vi "Delete_Fake_Dots_From_Array([-1,-1...]).vi"(2 "error IN":errorcluster, 3 "[IN] Source Array":dbl[][](array[numeric])) -> (0 "error OUT":errorcluster, 1 "[OUT] Filtered Array (X,Y,dX,dY)":dbl[][](array[numeric]))   [LabVIEW 2017]
doc: "Getting rid of deleted displacements (-1,-1,...)"
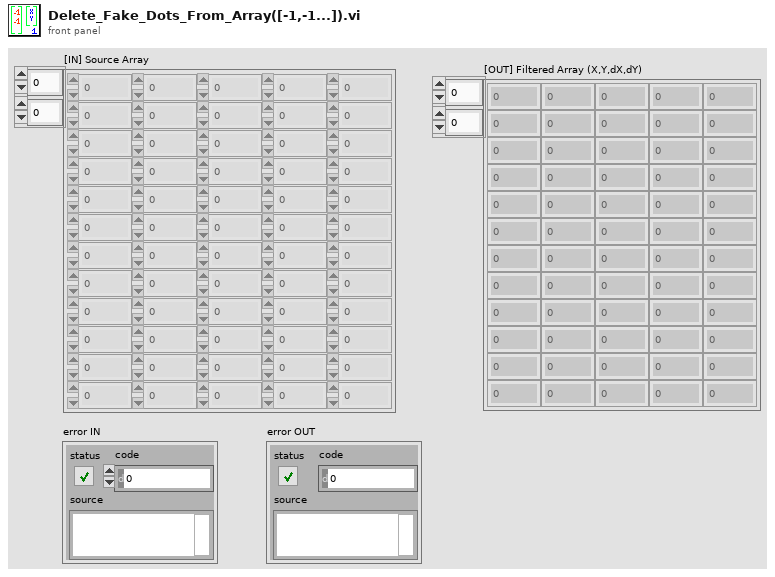
[diagram p1: front panel]
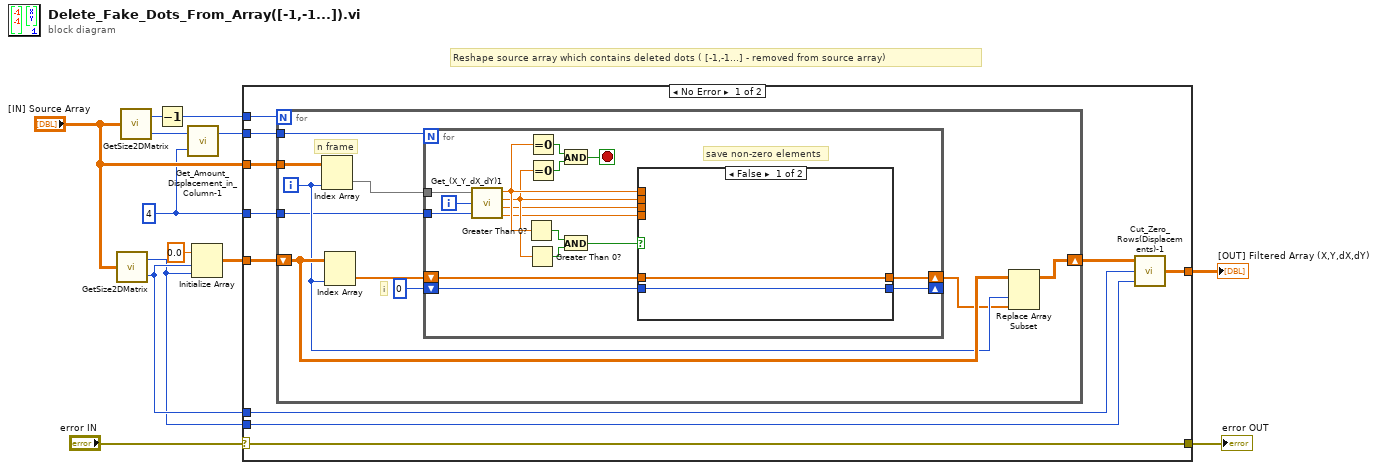
[diagram p0: block diagram]
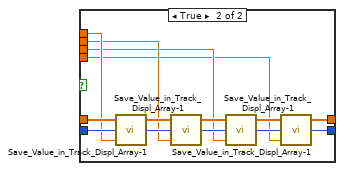
[diagram p2: hidden frame]
diagram:
  w3 = 4 ("y")
  # "Reshape source array which contains deleted dots ( [-1,-1...] - removed from source array)"
  n1 = call "GetSize2DMatrix.vi"("Array IN (2D)"="[IN] Source Array") -> ("# Cols"=w7:i32, "# Rows"=w8:i32)
  n2 = call "GetSize2DMatrix.vi"("Array IN (2D)"="[IN] Source Array") -> ("# Cols"=w13:i32, "# Rows"=w5:i32)
  n3 = Decrement(x=w13) -> (x-1=w12:i32)
  n4 = call "Get_Amount_Displacement_in_Column-1.vi"("multiplier"=w3, "# Rows"=w5) -> ("Displ amount"=w4:i32)  [unwired: 1 out]
  n5 = Initialize Array(0.0 ("element"), w8, w7) -> (w9:dbl[][])
  n6 = case shown="No Error" "error IN" {
    selector: "error IN" -> [w14 w67]
    tunnel: w12 -> [w23 _]
    tunnel: "[IN] Source Array" -> [w22 _]
    tunnel: w9 -> [w21 w68]
    tunnel: w8 -> [w19 _]
    tunnel: w7 -> [w18 _]
    tunnel: [w17 w68] -> w6
    tunnel: w4 -> [w16 _]
    tunnel: w3 -> [w15 _]
    tunnel: [w14 w67] -> w1
    frame No Error {
      n7 = for {
        N: w23 -> [_]
        tunnel: w22 -> [w33]
        shift-right: [w29] -> w20
        shift-left: w21 -> [w30]
        tunnel: w16 -> [w25]
        tunnel: w15 -> [w24]
        i -> [w28]
        # "i"
        # "n frame"
        n8 = Index Array(array=w33, index (col)=w28) -> (element=w31:dbl[])  [unwired: 1 in]
        n9 = Index Array(array=w30, index (col)=w28) -> (element=w26:dbl[])  [unwired: 1 in]
        n10 = for {
          N: w25 -> [_]
          tunnel: w31 -> [w50]
          tunnel: w24 -> [w48]
          shift-right: [w34] -> w27
          shift-left: w26 -> [w41]
          shift-right: [w35] -> _
          shift-left: 0 -> [w40]
          i -> [w49]
          stop <- w45 stop-if-true
          # "save non-zero elements"
          n11 = call "Get_(X_Y_dX_dY)1.vi"("(X,Y,dX,dY)"=w50, "index"=w49, "multiplier"=w48) -> ("X"=w39:dbl, "Y"=w38:dbl, "dX"=w37:dbl, "dY"=w36:dbl)
          n12 = Greater Than 0?(x=w39) -> (x > 0?=w44:bool)
          n13 = Greater Than 0?(x=w38) -> (x > 0?=w43:bool)
          n14 = Equal To 0?(x=w39) -> (x = 0?=w47:bool)
          n15 = Equal To 0?(x=w38) -> (x = 0?=w46:bool)
          n16 = And(x=w47, y=w46) -> (x .and. y?=w45:bool)
          n17 = And(x=w44, y=w43) -> (x .and. y?=w42:bool)
          n18 = case shown="False" w42 {
            tunnel: w41 -> [w52 w66]
            tunnel: w40 -> [w51 w65]
            tunnel: w39 -> [_ w64]
            tunnel: w38 -> [_ w61]
            tunnel: w37 -> [_ w58]
            tunnel: w36 -> [_ w55]
            tunnel: [w51 w53] -> w35
            tunnel: [w52 w54] -> w34
            frame False {
            }
            frame True {
              n19 = call "Save_Value_in_Track_Displ_Array-1.vi"("[IN] Value"=w64, "[IN] Index"=w65, "[IN] Empty tracks\nfor points saving"=w66) -> ("[OUT] Index ++"=w62:i32, "[OUT Track with saved value"=w63:dbl[])  [unwired: 1 in]
              n20 = call "Save_Value_in_Track_Displ_Array-1.vi"("[IN] Value"=w61, "[IN] Index"=w62, "[IN] Empty tracks\nfor points saving"=w63) -> ("[OUT] Index ++"=w59:i32, "[OUT Track with saved value"=w60:dbl[])  [unwired: 1 in]
              n21 = call "Save_Value_in_Track_Displ_Array-1.vi"("[IN] Value"=w58, "[IN] Index"=w59, "[IN] Empty tracks\nfor points saving"=w60) -> ("[OUT] Index ++"=w56:i32, "[OUT Track with saved value"=w57:dbl[])  [unwired: 1 in]
              n22 = call "Save_Value_in_Track_Displ_Array-1.vi"("[IN] Value"=w55, "[IN] Index"=w56, "[IN] Empty tracks\nfor points saving"=w57) -> ("[OUT] Index ++"=w53:i32, "[OUT Track with saved value"=w54:dbl[])  [unwired: 1 in]
            }
          }
        }
        n23 = Replace Array Subset(array=w30, new element=w27, index (col)=w28) -> (w29:dbl[][])  [unwired: 1 in]
      }
      n24 = call "Cut_Zero_Rows(Displacements)-1.vi"("# Cols"=w18, "# Rows"=w19, "Array IN"=w20) -> ("Array OUT"=w17:dbl[][])
    }
    frame Error {
    }
  }
  "[OUT] Filtered Array (X,Y,dX,dY)" <- w6
  "error OUT" <- w1
